vi "Unpack Panel Close.vi"(11 "PanelCloseMsg":refnum<class "PanelCloseMsg.lvclass">) -> (1 "Time":u32, 2 "VI Name":string, 3 "VI Refnum":refnum<vi>)   [LabVIEW 2017, in "ActorEvents.lvlib" / "PanelCloseMsg.lvclass"]
doc: "<License>\nCopyright © 2017 Composed Systems, LLC | All rights reserved\nwww.composed.io\n\nAuthor: Ethan Stern <ethan.stern@composed.io>\n\nThis software is provided \"AS IS\" WITHOUT WARRANTIES, either express or implied, AND IS FOR EDUCATIONAL PURPOSES ONLY.\n</License>"
uses:
  PanelCloseMsg.lvclass
  PanelCloseMsg.lvclass/PanelCloseMsg.ctl
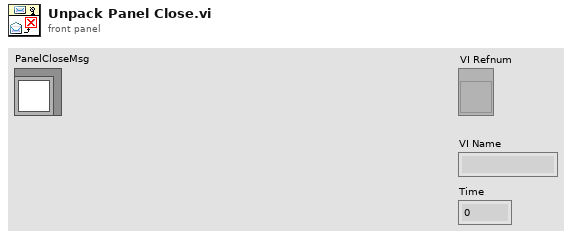
[diagram p1: front panel]
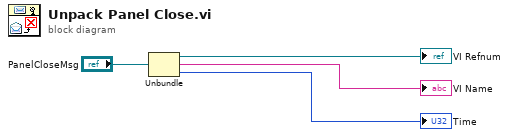
[diagram p0: block diagram]
diagram:
  n1 = Unbundle("PanelCloseMsg") -> (→"VI Refnum":refnum<vi>, →"VI Name":string, →"Time":u32)
